vi "KeDSO Abort Digitizing Process.vi"(8 "error in":errorcluster, 11 "keysight dso":T1 {"bw limit [Hz]" format="%#_6p"; "channels"."Offset [V]" min=0.0 format="%#_6p"; "channels"."Range [Vpk]" min=0.0 format="%#_6p"; "channels"."Channel" min=1}) -> (0 "error out":errorcluster, 3 "keysight dso out":T1 {"bw limit [Hz]" format="%#_6p"; "channels"."Offset [V]" min=0.0 format="%#_6p"; "channels"."Range [Vpk]" min=0.0 format="%#_6p"; "channels"."Channel" min=1})   [LabVIEW 2013]
doc: "Aborts current acquisition."
uses:
  KeDSO session.ctl
  KeDSO Virtual Channel.ctl
  KeDSO Trigger Setup.ctl
  KeDSO Trigger Source.ctl
  Agilent 90000 Series.lvlib
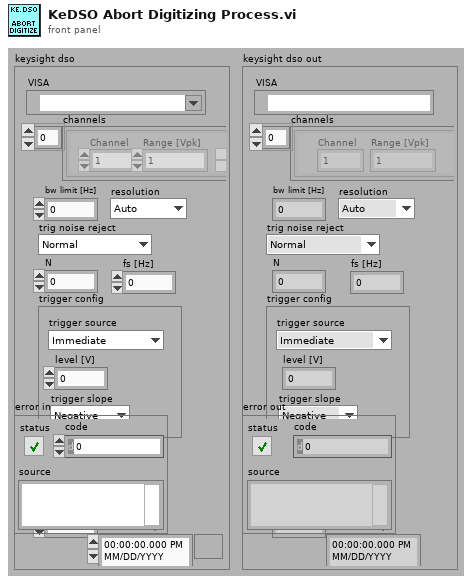
[diagram p1: front panel]
types:
  T1 = typedef "KeDSO session.ctl" = cluster{"VISA":refnum<visa-resource-name>, "channels":T2[], "bw limit [Hz]":dbl, "resolution":enum16{"Auto", "Bits 9", "Bits 10", "Bits 11", "Bits 12"}, "trig noise reject":enum16{"Normal", "High Sensitivity"}, "N":i64, "trigger config":T3, "fs [Hz]":dbl, "timeout stop":timestamp, "waiting for opc":bool, "fetch offset [smpl]":i64, "abs timestamp":timestamp}
  T2 = typedef "KeDSO Virtual Channel.ctl" = cluster{"Channel":i32, "Range [Vpk]":dbl, "btn clr":bool, "btn up":bool, "btn down":bool, "Offset [V]":dbl, "Coupling":enum16{"DC", "DC50", "AC", "LFR1"}, "bw limit enab":bool}
  T3 = typedef "KeDSO Trigger Setup.ctl" = cluster{"trigger source":T4, "level [V]":dbl, "trigger slope":enum16{"Negative", "Positive", "Either"}}
  T4 = typedef "KeDSO Trigger Source.ctl" = enum16{"Immediate", "Level", "AUX"}
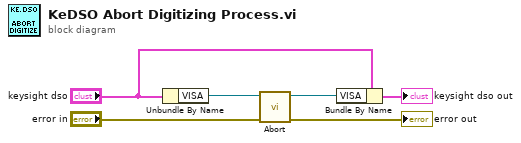
[diagram p0: block diagram]
diagram:
  n1 = Unbundle By Name("keysight dso") -> ("VISA"=w2:refnum<visa-resource-name>)
  n2 = call "Abort.vi"("error in (no error)"="error in", "VISA resource name"=w2) -> ("error out"=→"error out":errorcluster, "VISA resource name out"=w1:refnum<visa-resource-name>)  [unwired: 8 in]
  n3 = Bundle By Name(cluster="keysight dso", "VISA"=w1) -> (→"keysight dso out":T1)
